vi "Create.vi"() -> (7 "Role Manager Identity out":refnum<class "Role Manager Identity.lvclass">)   [LabVIEW 2020, in "Volatus.lvlib" / "Role Manager Identity.lvclass"]
uses:
  Role Manager Identity.lvclass
  Role Manager Identity.lvclass/Role Manager Identity.ctl
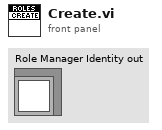
[diagram p1: front panel]
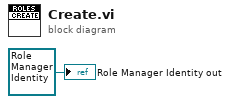
[diagram p0: block diagram]
diagram:
  "Role Manager Identity out" <- refnum<class "Role Manager Identity.lvclass"> refnum ("Role Manager Identity out")
